vi "DSF.Memory.Pointer.I32.Read.0D.vi"(8 "error in (no error)":errorcluster, 9 "offset (0)":u64 format="%d bytes", 10 "value in":i32, 11 "pointer in":refnum<class "DSF.Memory.Pointer.I32.lvclass">) -> (0 "error out":errorcluster, 1 "offset out":u64 format="%d bytes", 2 "value out":i32, 3 "pointer out":refnum<class "DSF.Memory.Pointer.I32.lvclass">)   [LabVIEW 2016, in "DSF.Memory.lvlib" / "DSF.Memory.Pointer.I32.lvclass"]
uses:
  DSF.Memory.Pointer.I32.lvclass
  C:/Git/SourceTree/data-sharing-framework/Source/Submodules/Memory Manager/Source/Classes/Pointer/Memory.Pointer.lvclass
  Submodules/Memory Manager/Source/Classes/Pointer/Memory.Pointer.lvclass/Memory.Pointer.ctl
  Submodules/Memory Manager/Source/Classes/Pointer/Methods/Memory.Pointer.Read.Safe.0D.I32.vi
  Submodules/Memory Manager/Source/Classes/Pointer/Methods/Memory.Pointer.Read.Unsafe.0D.I32.vi
  Submodules/Memory Manager/Source/Classes/Pointer/Methods/Memory.Pointer.Parameter Check.Null Pointer.vi
  Submodules/Memory Manager/Source/Classes/Pointer/Methods/Memory.Pointer.Parameter Check.Subset.vi
  Submodules/Memory Manager/Source/Classes/Pointer/Accessors/Get Address.vi
  Submodules/Memory Manager/Source/Classes/Pointer/Methods/Memory.Pointer.Errors.vi
  Submodules/Memory Manager/Source/Classes/Pointer/Methods/Memory.Pointer.Errors.Null Pointer.vi
  Submodules/Memory Manager/Source/Classes/Pointer/Methods/Memory.Pointer.Errors.Out of Bounds.vi
  Submodules/Memory Manager/Source/Classes/Pointer/Accessors/Get Size.vi
  Submodules/Memory Manager/Source/Classes/Pointer/Methods/Memory.Pointer.Errors.Create Error.vi
  Submodules/Memory Manager/Source/Submodules/SEH/Source/VIs/Static Error Handling.Source Buffer.Write.String.vi
  Submodules/Memory Manager/Source/Classes/Pointer/Methods/Memory.Pointer.Errors.Write Pointer Size.vi
  Submodules/Memory Manager/Source/Submodules/SEH/Source/VIs/Static Error Handling.Source Buffer.Write.Numeric.Scalar.Base10.vi
  Submodules/Memory Manager/Source/Submodules/SEH/Source/VIs/Static Error Handling.Source Buffer.Write.Numeric.Scalar.Base10 (U64).vi
  Submodules/Memory Manager/Source/Submodules/SEH/Source/VIs/Static Error Handling.Error Cluster Constant.vi
  Submodules/Memory Manager/Source/Submodules/SEH/Source/VIs/Static Error Handling.Error Cluster Constant (256B).vi
  Submodules/Memory Manager/Source/Submodules/SEH/Source/VIs/Static Error Handling.Parameters.Status.Set.vi
  Submodules/Memory Manager/Source/Submodules/SEH/Source/VIs/Static Error Handling.Parameters.Code.Set.vi
  Submodules/Memory Manager/Source/Submodules/SEH/Source/VIs/Static Error Handling.Parameters.VI Source.Set.vi
  Submodules/Memory Manager/Source/Constants/Memory.Constants.vi
  Submodules/Memory Manager/Source/Constants/Memory.Constants.Library Name.vi
  Submodules/Memory Manager/Source/Classes/Pointer/Methods/Memory.Pointer.Errors.Get Info.vi
  Submodules/Memory Manager/Source/Classes/Pointer/Memory.Pointer.lvclass
  C:/Git/SourceTree/data-sharing-framework/Source/Submodules/Memory Manager/Source/Classes/Pointer.Internal/Memory.Pointer.Internal.lvclass
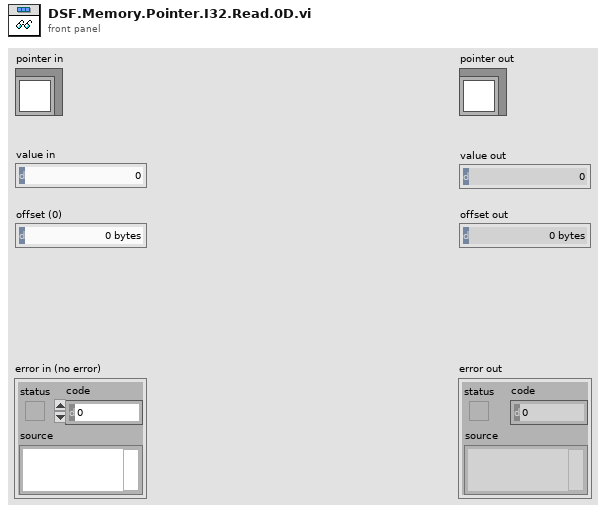
[diagram p1: front panel]
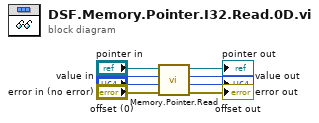
[diagram p0: block diagram]
diagram:
  n1 = call-poly "Memory.Pointer.Read.vi"("error in (no error)"="error in (no error)", "offset (0)"="offset (0)", "value in"="value in", "pointer in"="pointer in") -> ("error out"=→"error out":errorcluster, "offset out"=→"offset out":u64, "value out"=→"value out":i32, "pointer out"=→"pointer out":refnum<class "DSF.Memory.Pointer.I32.lvclass">)  [unwired: 4 in]
